vi "init_Kloehn.vi"(1 "kloehn session in":T1={"VISA resource out"="COM12", "error out"={"status"=FALSE, "code"=0, "source"=""}}) -> (0 "kloehn session out":T1={"VISA resource out"="COM12", "error out"={"status"=FALSE, "code"=0, "source"=""}})   [LabVIEW 2010]
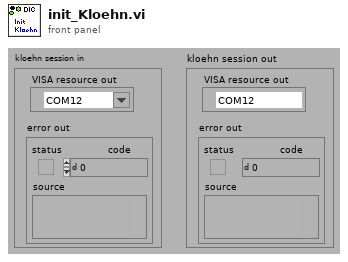
[diagram p1: front panel]
types:
  T1 = cluster{"VISA resource out":refnum<visa-resource-name>, "error out":errorcluster}
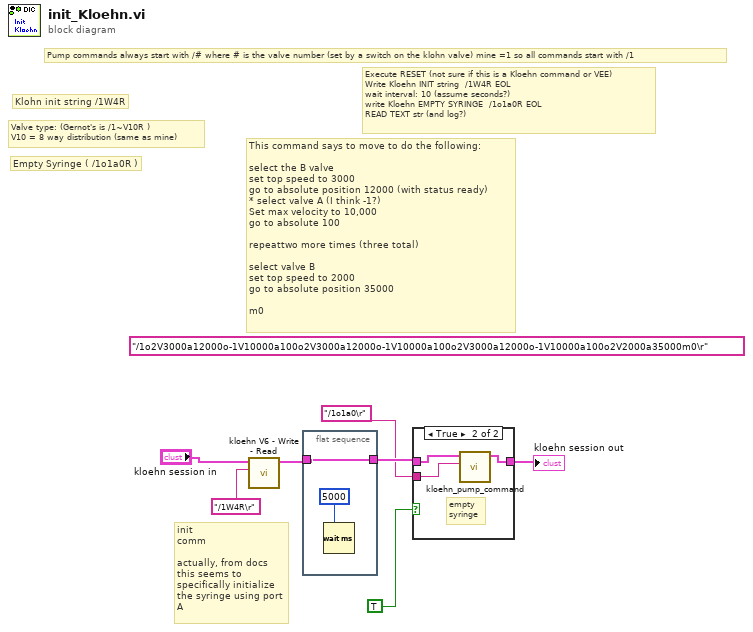
[diagram p0: block diagram]
diagram:
  (unwired) "/1o2V3000a12000o-1V10000a100o2V3000a12000o-1V10000a100o2V3000a12000o-1V10000a100o2V2000a35000m0\r"
  # "This command says to move to do the following:\n\nselect the B valve\nset top speed to 3000\ngo to absolute position 12000 (with status ready)\n* select valve A (I think -1?)\nSet max velocity to 10,000\ngo to absolute 100\n\nrepeattwo more times (three total)\n\nselect valve B\nset top speed to 2000\ngo to absolute position 35000\n\nm0"
  # "init\ncomm\n\nactually, from docs this seems to specifically initialize the syringe using port A"
  # "Pump commands always start with /# where # is the valve number (set by a switch on the klohn valve) mine =1 so all commands start with /1"
  # "Execute RESET (not sure if this is a Kloehn command or VEE)\nWrite Kloehn INIT string  /1W4R EOL\nwait interval: 10 (assume seconds?)\nwrite Kloehn EMPTY SYRINGE  /1o1a0R EOL\nREAD TEXT str (and log?)"
  # "Empty Syringe ( /1o1a0R )"
  # "Valve type: (Gernot's is /1~V10R )\nV10 = 8 way distribution (same as mine)"
  # "Klohn init string /1W4R"
  n1 = call "kloehn V6 - Write - Read.vi"("Send String"="/1W4R\r", "kloehn session in"="kloehn session in") -> ("kloehn session out"=w5:T1)  [unwired: 6 in, 3 out]
  n2 = flat-sequence {
    tunnel: w5 -> [w9]
    tunnel: [w9] -> w6
    frame #0 {
      n3 = Wait (ms)(milliseconds to wait=5000) -> ()  [unwired: 1 out]
    }
  }
  n4 = case shown="True" TRUE {
    tunnel: w6 -> [w10 w13]
    tunnel: [w10 w11] -> w1
    tunnel: "/1o1a0\r" ("Send String") -> [_ w12]
    frame False {
    }
    frame True {
      # "empty\nsyringe"
      n5 = call "kloehn_pump_command.vi"("Send String"=w12, "kloehn session in"=w13) -> ("kloehn session out"=w11:T1)  [unwired: 6 in, 3 out]
    }
  }
  "kloehn session out" <- w1
